vi "top_level.vi"() -> ()   [LabVIEW 2014]
panel:
  in  "C_____F":bool
  in  "Summer___Winter":bool
  out "Waveform Chart":dbl(graph)
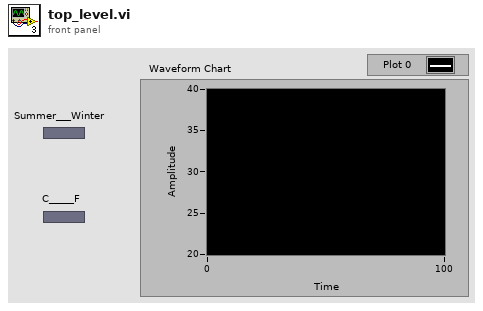
[diagram p1: front panel]
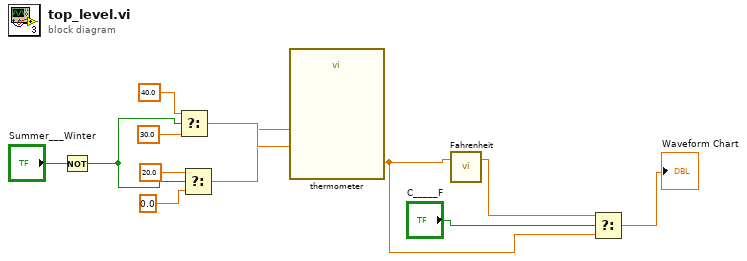
[diagram p0: block diagram]
diagram:
  n1 = Not(x="Summer___Winter") -> (.not. x?=w1:bool)
  n2 = Select(t=40.0, s=w1, f=30.0) -> (s? t:f=w8:dbl)
  n3 = Select(t=20.0, s=w1, f=0.0) -> (s? t:f=w7:dbl)
  n4 = call "thermometer.vi"("lower_bound"=w7, "upper_bound"=w8) -> ("Numeric"=w6:dbl)  [unwired: 2 in]
  n5 = call "Fahrenheit.vi"("C"=w6) -> ("F"=w5:dbl)  [unwired: 2 in]
  n6 = Select(t=w5, s="C_____F", f=w6) -> (s? t:f=→"Waveform Chart":dbl)
